vi "Configure EPICS Server - Host.vi"() -> ()   [LabVIEW 2011]
uses:
  <vilib>/lvdsc/process/internal/data type.ctl
  <vilib>/variable/tagger/epicsserver/API/internal/Undeploy EPICS Server (By Ref).vi
  <vilib>/variable/tagger/epicsserver/API/internal/EPICSServerClass/EPICSServer.lvclass
  <vilib>/variable/tagger/epicsserver/API/NI_EPICS_Server.lvlib
  Program Files (x86)/National Instruments/LabVIEW 2011/resource/objmgr/ni.var.rc
panel:
  out "URL":string
  out "EPICS Server Attributes":T2(array[cluster])
  in  "Delete":bool
  in  "Create/Update":bool
  in  "Custom PV name (Optional)":string
  in  "Variable path":refnum<k21>="ni.var.psp://localhost/HostSource/VarDouble"
  in  "Source process":refnum<k21>="ni.var.psp://localhost/HostSource"
  in  "Create All":bool
  in  "Stop":bool
  in  "Create EPICS server on":string(combo)="localhost"
  # "Publish all shared varaibles under the process as PVs"
  # "EPICS server attributes:"
  # "PV name"
  # "Variable path"
  # "Data type"
  # "Access type"
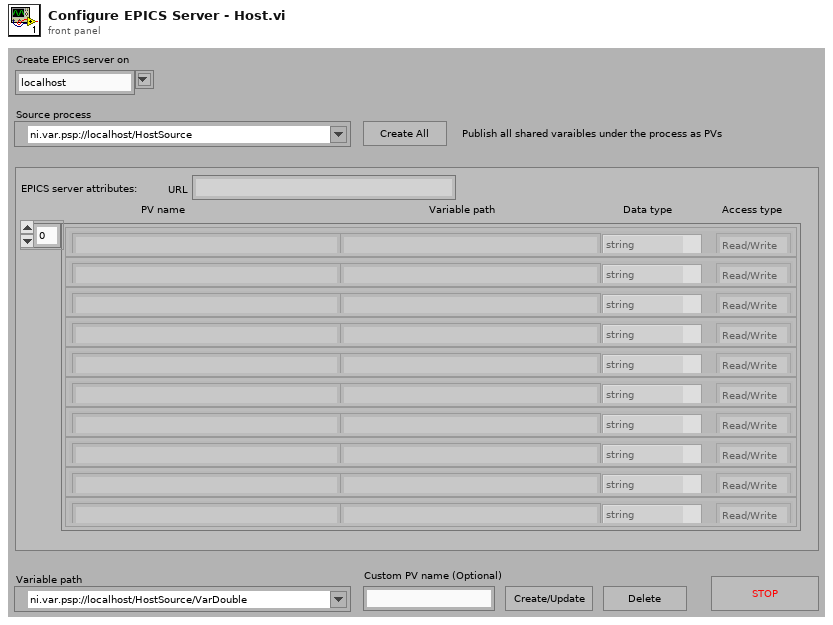
[diagram p1: front panel]
types:
  T1 = typedef "data type.ctl" = enum32{"u32BitField", "bool", "double", "string", "int8", "uint8", "int16", "uint16", "int32", "uint32", "int64", "uint64", "single", "double waveform", "int16 waveform", "array of boolean", "array of int8", "array of uint8", "array of int16", "array of uint16", "array of int32", "array of uint32", "array of int64", "array of uint64", "array of single", "array of double", "array of double waveform", "array of int16 waveform", "array of string", "variant", "timestamp", "fixed point", "custom"}
  T2 = cluster{"PV name":string, "variable path":string, "data type":T1, "access type":enum16{"Read/Write", "Read Only"}}[]
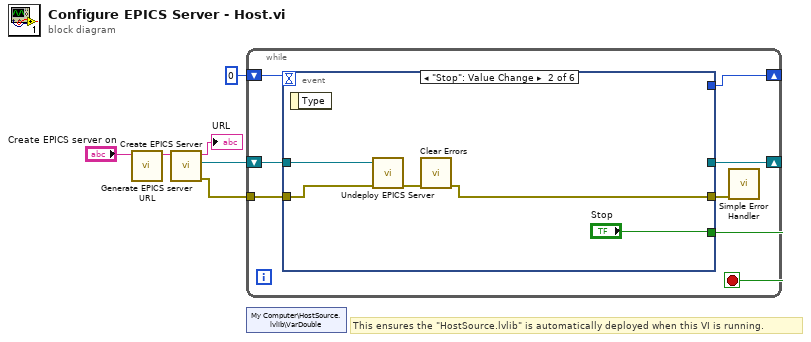
[diagram p0: block diagram]
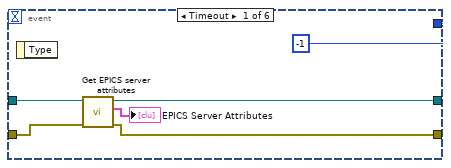
[diagram p2: hidden frame]
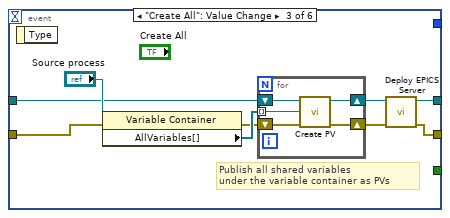
[diagram p3: hidden frame]
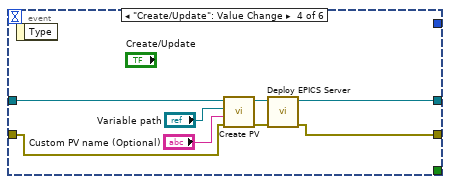
[diagram p4: hidden frame]
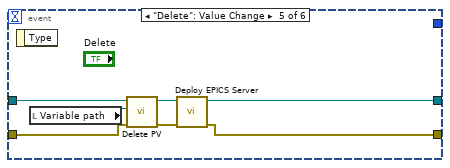
[diagram p5: hidden frame]
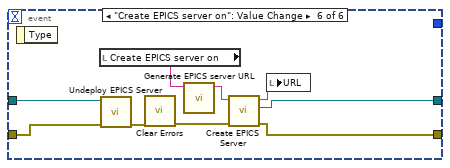
[diagram p6: hidden frame]
diagram:
  # "This ensures the \"HostSource.lvlib\" is automatically deployed when this VI is running."
  n1 = call "Generate EPICS server URL.vi"("machine"="Create EPICS server on") -> ("EPICS server URL"=w4:string)  [unwired: 10 in]
  n2 = call <vilib>:"Create EPICS Server.vi"("EPICS Server URL in"=w4) -> ("error out"=w1:errorcluster, "EPICS Server ref"=w2:refnum<data-value>, "EPICS Server URL out"=→"URL":string)  [unwired: 8 in]
  n3 = while {
    shift-right: [w11] -> _
    shift-left: w2 -> [w12]
    shift-right: [w9] -> _
    shift-left: 0 -> [w10]
    tunnel: w1 -> [w8]
    stop <- w13 stop-if-true
    n4 = event shown="[1] \"Stop\": Value Change" {
      selector: _ -> [_ _ _ _ _ _]
      dyn-events: _ -> [_ _ _ _ _ _]
      timeout: w10 -> [_ _ _ _ _ _]
      tunnel: [_ "Stop" _ _ _ _] -> w13
      tunnel: w12 -> [w18 w23 w31 w46 w52 w61]
      tunnel: [w17 _ w29 w42 w50 w56] -> w11
      tunnel: [-1 _ _ _ _ _] -> w9
      tunnel: w8 -> [w15 w21 w27 w40 w48 w55]
      tunnel: [w14 w20 w25 w39 w47 w54] -> w7
      event Timeout {
        n5 = event-data() -> ()  [unwired: 1 in, 1 out]
        n6 = call "Get EPICS server attributes.vi"("error in (no error)"=w15, "EPICS server ref in"=w18) -> ("error out"=w14:errorcluster, "EPICS server attributes"=→"EPICS Server Attributes":T2, "EPICS server ref out"=w17:refnum<data-value>)  [unwired: 7 in]
      }
      event "Stop": Value Change {
        n7 = event-data() -> ()  [unwired: 1 in, 1 out]
        n8 = call-poly <vilib>:"Undeploy EPICS Server.vi"("error in (no error)"=w21, "EPICS Server ref"=w23) -> ("error out"=w22:errorcluster)  [unwired: 9 in]
        n9 = call <vilib>:"Clear Errors.vi"("error in (no error)"=w22) -> ("error out"=w20:errorcluster)  [unwired: 6 in]
      }
      event "Create All": Value Change {
        # "Publish all shared variables\nunder the variable container as PVs"
        n10 = event-data() -> ()  [unwired: 1 in, 1 out]
        n11 = property class="Variable Container"(reference="Source process", error in=w27) -> (error out=w26:errorcluster, "AllVariables[]"=w33:refnum<k21>[])  [unwired: 1 out]
        n12 = for {
          tunnel: w33 -> [w37] mode=indexing
          shift-right: [w34] -> w28
          shift-left: w26 -> [w35]
          shift-right: [w36] -> w30
          shift-left: w31 -> [w38]
          n13 = call <vilib>:"Create PV.vi"("error in (no error)"=w35, "variable path"=w37, "EPICS Server ref in"=w38) -> ("error out"=w34:errorcluster, "EPICS Server ref out"=w36:refnum<data-value>)  [unwired: 7 in]
        }
        n14 = call <vilib>:"Deploy EPICS Server.vi"("error in (no error)"=w28, "EPICS Server ref in"=w30) -> ("error out"=w25:errorcluster, "EPICS Server ref out"=w29:refnum<data-value>)  [unwired: 8 in]
      }
      event "Create/Update": Value Change {
        n15 = event-data() -> ()  [unwired: 1 in, 1 out]
        n16 = call <vilib>:"Create PV.vi"("error in (no error)"=w40, "PV name"="Custom PV name (Optional)", "variable path"="Variable path", "EPICS Server ref in"=w46) -> ("error out"=w41:errorcluster, "EPICS Server ref out"=w44:refnum<data-value>)  [unwired: 6 in]
        n17 = call <vilib>:"Deploy EPICS Server.vi"("error in (no error)"=w41, "EPICS Server ref in"=w44) -> ("error out"=w39:errorcluster, "EPICS Server ref out"=w42:refnum<data-value>)  [unwired: 8 in]
      }
      event "Delete": Value Change {
        n18 = event-data() -> ()  [unwired: 1 in, 1 out]
        n19 = local read "Variable path"() -> (w51:refnum<k21>)
        n20 = call <vilib>:"Delete PV.vi"("error in (no error)"=w48, "PV name or variable path"=w51, "EPICS Server ref in"=w52) -> ("error out"=w49:errorcluster, "EPICS Server ref out"=w53:refnum<data-value>)  [unwired: 7 in]
        n21 = call <vilib>:"Deploy EPICS Server.vi"("error in (no error)"=w49, "EPICS Server ref in"=w53) -> ("error out"=w47:errorcluster, "EPICS Server ref out"=w50:refnum<data-value>)  [unwired: 8 in]
      }
      event "Create EPICS server on": Value Change {
        n22 = event-data() -> ()  [unwired: 1 in, 1 out]
        n23 = local read "Create EPICS server on"() -> (w58:string)
        n24 = call-poly <vilib>:"Undeploy EPICS Server.vi"("error in (no error)"=w55, "EPICS Server ref"=w61) -> ("error out"=w60:errorcluster)  [unwired: 9 in]
        n25 = call <vilib>:"Clear Errors.vi"("error in (no error)"=w60) -> ("error out"=w59:errorcluster)  [unwired: 6 in]
        n26 = call "Generate EPICS server URL.vi"("machine"=w58) -> ("EPICS server URL"=w57:string)  [unwired: 10 in]
        n27 = call <vilib>:"Create EPICS Server.vi"("error in (no error)"=w59, "EPICS Server URL in"=w57) -> ("error out"=w54:errorcluster, "EPICS Server ref"=w56:refnum<data-value>, "EPICS Server URL out"=w62:string)  [unwired: 7 in]
        n28 = local write "URL"(w62) -> ()
      }
    }
    n29 = call <vilib>:"Simple Error Handler.vi"("error in (no error)"=w7) -> ()  [unwired: 4 in, 5 out]
  }
  n30 = shared-variable "My Computer\\HostSource.lvlib\\VarDouble"() -> ()  [unwired: 1 in, 2 out]
